vi "Tosca-Set Live AI Controls.vi"(0 "state":T2, 11 "Auto":refnum<vi>, 12 "Vscale":refnum<vi>, 13 "Trace":refnum<vi>) -> (8 "Controls":T1)   [LabVIEW 2020]
uses:
  Typedefs/Tosca-AI UI State.ctl
  Typedefs/Tosca-AI Plot Properties.ctl
  Typedefs/Tosca-AI Live Controls.ctl
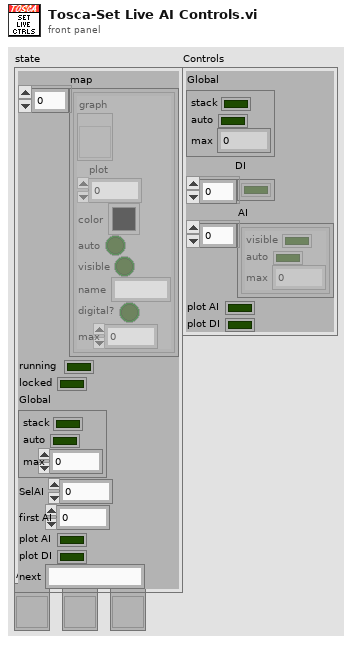
[diagram p1: front panel]
types:
  T1 = typedef "Tosca-AI Live Controls.ctl" = cluster{"Global":cluster{"stack":bool, "auto":bool, "max":dbl}, "DI":bool[], "AI":cluster{"visible":bool, "auto":bool, "max":dbl}[], "plot AI":bool, "plot DI":bool}
  T2 = typedef "Tosca-AI UI State.ctl" = cluster{"map":T3[], "running":bool, "locked":bool, "Global":cluster{"stack":bool, "auto":bool, "max":dbl}, "SelAI":i32, "first AI":i32, "plot AI":bool, "plot DI":bool, "next":string}
  T3 = typedef "Tosca-AI Plot Properties.ctl" = cluster{"graph":refnum<vi>, "plot":i32, "color":u32, "auto":bool, "visible":bool, "name":string, "digital?":bool, "max":dbl}
  T4 = enum8{"Enabled", "Disabled", "Disabled and Grayed Out"}
  T5 = cluster{"Global":cluster{"stack":bool, "auto":bool, "max":dbl}, bool[], cluster{"visible":bool, "auto":bool, "max":dbl}[], "plot AI":bool, "plot DI":bool}
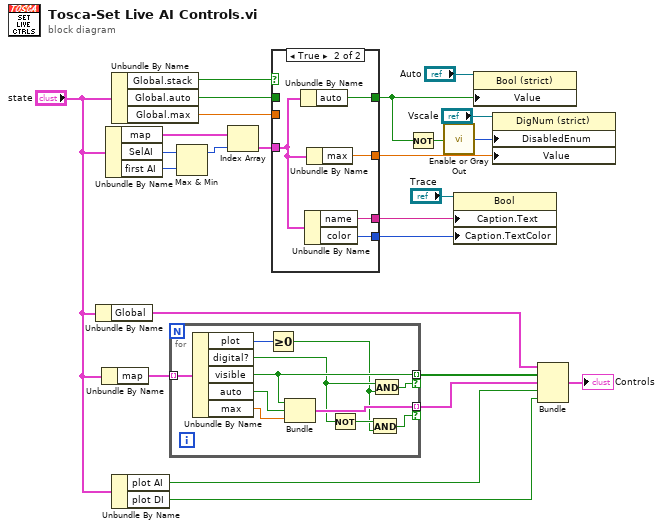
[diagram p0: block diagram]
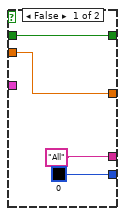
[diagram p2: hidden frame]
diagram:
  n1 = Unbundle By Name("state") -> ("Global"=w11:cluster{"stack":bool, "auto":bool, "max":dbl})
  n2 = Unbundle By Name("state") -> ("map"=w13:T3[])
  n3 = Unbundle By Name("state") -> ("map"=w7:T3[], "SelAI"=w6:i32, "first AI"=w5:i32)
  n4 = Unbundle By Name("state") -> ("Global.stack"=w25:bool, "Global.auto"=w20:bool, "Global.max"=w18:dbl)
  n5 = Unbundle By Name("state") -> ("plot AI"=w2:bool, "plot DI"=w1:bool)
  n6 = for {
    tunnel: w13 -> [w28] mode=indexing
    tunnel: [w36] -> w12 mode=indexing if=w31
    tunnel: [w34] -> w9 mode=indexing if=w26
    n7 = Unbundle By Name(w28) -> ("plot"=w33:i32, "digital?"=w32:bool, "visible"=w36:bool, "auto"=w35:bool, "max"=w27:dbl)
    n8 = Greater Or Equal To 0?(x=w33) -> (x >= 0?=w29:bool)
    n9 = Bundle("visible"=w36, "auto"=w35, "max"=w27) -> (w34:cluster{"visible":bool, "auto":bool, "max":dbl})  [unwired: 1 in]
    n10 = Not(x=w32) -> (.not. x?=w30:bool)
    n11 = And(x=w30, y=w29) -> (x .and. y?=w26:bool)
    n12 = And(x=w32, y=w29) -> (x .and. y?=w31:bool)
  }
  n13 = Max & Min(x=w6, y=w5) -> (max(x,y)=w4:i32)  [unwired: 1 out]
  n14 = Index Array(array=w7, index=w4) -> (element=w8:T3)
  n15 = case shown="True" w25 {
    tunnel: ["All" ("Caption.Text") w42] -> w23
    tunnel: [u32 0 w41] -> w22
    tunnel: [w38 w45] -> w14
    tunnel: w20 -> [w38 _]
    tunnel: [w37 w44] -> w17
    tunnel: w18 -> [w37 _]
    tunnel: w8 -> [_ w43]
    frame False {
    }
    frame True {
      n16 = Unbundle By Name(w43) -> ("auto"=w45:bool)
      n17 = Unbundle By Name(w43) -> ("name"=w42:string, "color"=w41:u32)
      n18 = Unbundle By Name(w43) -> ("max"=w44:dbl)
    }
  }
  n19 = Not(x=w14) -> (.not. x?=w15:bool)
  n20 = call "Enable or Gray Out.vi"("Boolean"=w15) -> ("Disabled"=w16:T4)
  n21 = property class="Bool"(reference="Trace", "Caption.Text"=w23, "Caption.TextColor"=w22) -> ()  [unwired: 1 in, 2 out]
  n22 = property class="Bool (strict)"(reference="Auto", "Value"=w14) -> ()  [unwired: 1 in, 2 out]
  n23 = property class="DigNum (strict)"(reference="Vscale", "DisabledEnum"=w16, "Value"=w17) -> ()  [unwired: 1 in, 2 out]
  n24 = Bundle("Global"=w11, w12, w9, "plot AI"=w2, "plot DI"=w1) -> (→"Controls":T5)  [unwired: 1 in]
